vi "MouseMove.vi"(7 "Buffer":refnum<queue>, 8 "error in":errorcluster, 9 "Coords":T5, 11 "Data in":T1={"Class"={"Ants"=refnum, "Layer"=refnum, "Templates"=refnum, "Icon"=refnum, "Glyph"=refnum, "Settings"=refnum, "Tools"=refnum}, "Ref"={"Add Layer"=refnum, "Remove Layer"=refnum, "Line Text"=[], "Body Text Spec"=refnum, "DNL_Font"=refnum, "glyph path str"=refnum, "templates path str"=refnum, "Arrow Up"=refnum, "Arrow Down"=refnum, "IE VI Ref"=refnum, "Glyphs tree"=refnum, "Templates tree"=refnum, "Layer Icon Text"=refnum, "Layer Template"=refnum, "Body Text"=refnum, "Search Templates"=refnum, "TextMarker"=refnum, "Tab Control"=refnum, "Search Glyphs"=refnum, "Line Color"=refnum, "DNL_Glyphs []"=refnum, "Fill Color"=refnum, "Tools"=refnum, "Icon"=refnum, "Preview"=refnum, "Ants"=refnum, "Terminals"=refnum, "menu reference"=refnum, "LayerNames"=[], "GlyphLoadAnimation"=refnum, "TemplateLoadAnimation"=refnum, "refreshGlyphs"=refnum, "refreshTemplates"=refnum}, "Support"={"AntsRect"={"left"=0, "top"=0, "right"=0, "bottom"=0}, "Mouse Move Coords"={"Horizontal"=0, "Vertical"=0}, "Mouse Down Coords"={"Horizontal"=0, "Vertical"=0}, "Temp Coord"={"Horizontal"=0, "Vertical"=0}, "Action"=enum."Default", "Edge Color"=4914962, "Fill Color"=16860, "Mouse Down?"=FALSE, "Draft Mode?"=FALSE, "Temp Icon"=bytes[3102], "CTRL Pressed"=FALSE, "Move Selection?"=FALSE, "AntsRect Orig"={"left"=0, "top"=0, "right"=0, "bottom"=0}, "Text"="", "TM Set?"=FALSE, "Mouse inside icon?"=FALSE, "Tool (old value)"=0, "Pencil Move Color"=0, "Swap Colors?"=FALSE, "Shift pressed?"=FALSE}}) -> (0 "error out":errorcluster, 3 "Data out":T1={"Class"={"Ants"=refnum, "Layer"=refnum, "Templates"=refnum, "Icon"=refnum, "Glyph"=refnum, "Settings"=refnum, "Tools"=refnum}, "Ref"={"Add Layer"=refnum, "Remove Layer"=refnum, "Line Text"=[], "Body Text Spec"=refnum, "DNL_Font"=refnum, "glyph path str"=refnum, "templates path str"=refnum, "Arrow Up"=refnum, "Arrow Down"=refnum, "IE VI Ref"=refnum, "Glyphs tree"=refnum, "Templates tree"=refnum, "Layer Icon Text"=refnum, "Layer Template"=refnum, "Body Text"=refnum, "Search Templates"=refnum, "TextMarker"=refnum, "Tab Control"=refnum, "Search Glyphs"=refnum, "Line Color"=refnum, "DNL_Glyphs []"=refnum, "Fill Color"=refnum, "Tools"=refnum, "Icon"=refnum, "Preview"=refnum, "Ants"=refnum, "Terminals"=refnum, "menu reference"=refnum, "LayerNames"=[], "GlyphLoadAnimation"=refnum, "TemplateLoadAnimation"=refnum, "refreshGlyphs"=refnum, "refreshTemplates"=refnum}, "Support"={"AntsRect"={"left"=0, "top"=0, "right"=0, "bottom"=0}, "Mouse Move Coords"={"Horizontal"=0, "Vertical"=0}, "Mouse Down Coords"={"Horizontal"=0, "Vertical"=0}, "Temp Coord"={"Horizontal"=0, "Vertical"=0}, "Action"=enum."Default", "Edge Color"=4914962, "Fill Color"=16860, "Mouse Down?"=FALSE, "Draft Mode?"=FALSE, "Temp Icon"=bytes[3102], "CTRL Pressed"=FALSE, "Move Selection?"=FALSE, "AntsRect Orig"={"left"=0, "top"=0, "right"=0, "bottom"=0}, "Text"="", "TM Set?"=FALSE, "Mouse inside icon?"=FALSE, "Tool (old value)"=0, "Pencil Move Color"=0, "Swap Colors?"=FALSE, "Shift pressed?"=FALSE}})   [LabVIEW 2020]
uses:
  Class/Ants/Ants.lvclass
  Class/FakedArray/FakedArray.lvclass
  vi.lib/LabVIEW Icon API/lv_icon/Classes/Icon/Icon.lvclass
  Class/Icon Library/Glyph.lvclass
  Class/Settings/Settings.lvclass
  Class/Tools/Tools Paint.lvclass
  Controls/SupportClass_Action.ctl
  vi.lib/LabVIEW Icon API/lv_icon/lv_icon.lvlib
  <vilib>/Utility/miscctls.llb/LVPoint32TypeDef.ctl
  vi.lib/LabVIEW Icon API/lv_icon/Controls/IEColor.ctl
  Controls/SupportClass.ctl
  Controls/References Cluster.ctl
  Controls/IE Classes.ctl
  Controls/Global Data.ctl
panel:
  out "size(s)":i32
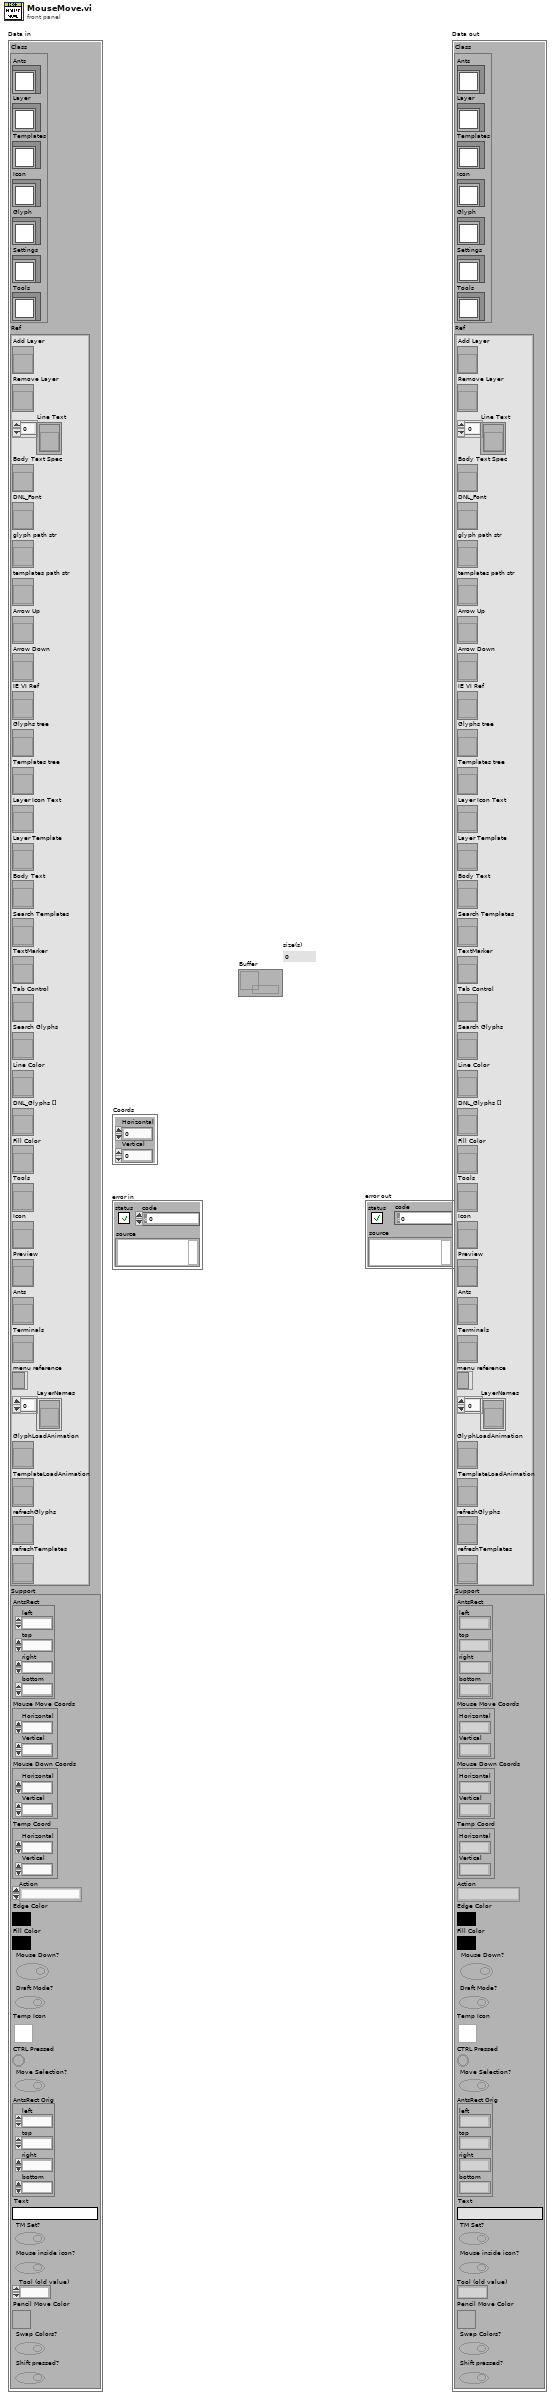
[diagram p1: front panel]
types:
  T1 = typedef "lv_icon.lvlib/Global Data.ctl" = cluster{"Class":T2, "Ref":T3, "Support":T4}
  T2 = typedef "IE Classes.ctl" = cluster{"Ants":refnum<class "Ants.lvclass">, "Layer":refnum<class "FakedArray.lvclass">, "Templates":refnum<class "FakedArray.lvclass">, "Icon":refnum<class "Icon.lvclass">, "Glyph":refnum<class "Glyph.lvclass">, "Settings":refnum<class "Settings.lvclass">, "Tools":refnum<class "Tools Paint.lvclass">}
  T3 = typedef "lv_icon.lvlib/References Cluster.ctl" = cluster{"Add Layer":refnum<vi>, "Remove Layer":refnum<vi>, "Line Text":refnum<vi>[], "Body Text Spec":refnum<vi>, "DNL_Font":refnum<vi>, "glyph path str":refnum<vi>, "templates path str":refnum<vi>, "Arrow Up":refnum<vi>, "Arrow Down":refnum<vi>, "IE VI Ref":refnum<vi>, "Glyphs tree":refnum<vi>, "Templates tree":refnum<vi>, "Layer Icon Text":refnum<vi>, "Layer Template":refnum<vi>, "Body Text":refnum<vi>, "Search Templates":refnum<vi>, "TextMarker":refnum<vi>, "Tab Control":refnum<vi>, "Search Glyphs":refnum<vi>, "Line Color":refnum<vi>, "DNL_Glyphs []":refnum<vi>, "Fill Color":refnum<vi>, "Tools":refnum<vi>, "Icon":refnum<vi>, "Preview":refnum<vi>, "Ants":refnum<vi>, "Terminals":refnum<vi>, "menu reference":refnum<k9>, "LayerNames":refnum<vi>[], "GlyphLoadAnimation":refnum<vi>, "TemplateLoadAnimation":refnum<vi>, "refreshGlyphs":refnum<vi>, "refreshTemplates":refnum<vi>}
  T4 = typedef "SupportClass.ctl" = cluster{"AntsRect":cluster{"left":i16, "top":i16, "right":i16, "bottom":i16}, "Mouse Move Coords":T5, "Mouse Down Coords":T5, "Temp Coord":T5, "Action":T6, "Edge Color":T7, "Fill Color":T7, "Mouse Down?":bool, "Draft Mode?":bool, "Temp Icon":picture, "CTRL Pressed":bool, "Move Selection?":bool, "AntsRect Orig":cluster{"left":i16, "top":i16, "right":i16, "bottom":i16}, "Text":string, "TM Set?":bool, "Mouse inside icon?":bool, "Tool (old value)":u32, "Pencil Move Color":u32, "Swap Colors?":bool, "Shift pressed?":bool}
  T5 = typedef "LVPoint32TypeDef.ctl" = cluster{"Horizontal":i32, "Vertical":i32}
  T6 = typedef "SupportClass_Action.ctl" = enum16{"Default", "Move Selection", "Glyph Library", "Tool"}
  T7 = typedef "IEColor.ctl" = u32
  T8 = cluster{"left":i16, "top":i16, "right":i16, "bottom":i16}
  T9 = typedef "Graphic.ctl" = cluster{"Rectangle":cluster{"left":i16, "top":i16, "right":i16, "bottom":i16}, "Path":path, "Image":picture, "Filter":string, "FileName":string}
  T10 = typedef "Tools.ctl" = enum32{"Pencil", "Line", "Dropper", "Fill", "Rectangle", "Filled Rectangle", "Ellipse", "Filled Ellipse", "Eraser", "Text", "Select", "Move"}
  T11 = cluster{"Horizontal":i32, "Vertical":i32, "Horizontal":i32, "Vertical":i32}
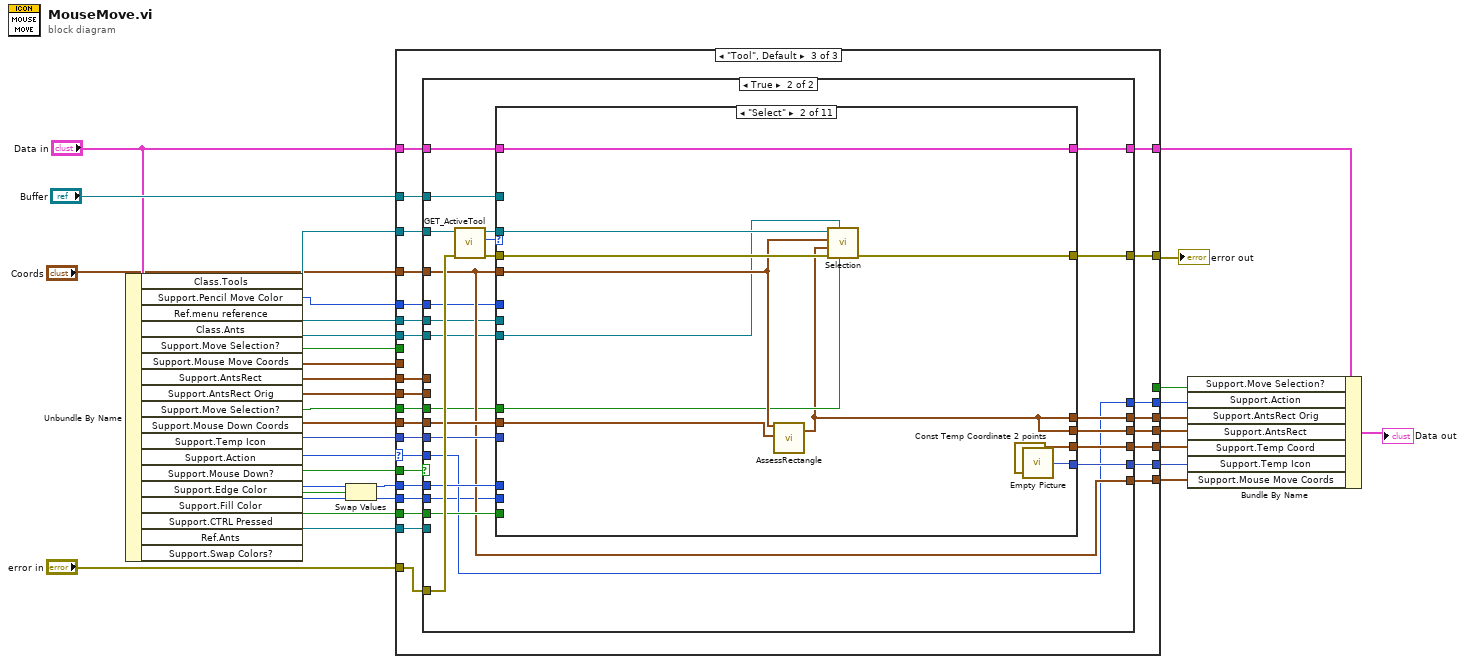
[diagram p0: block diagram]
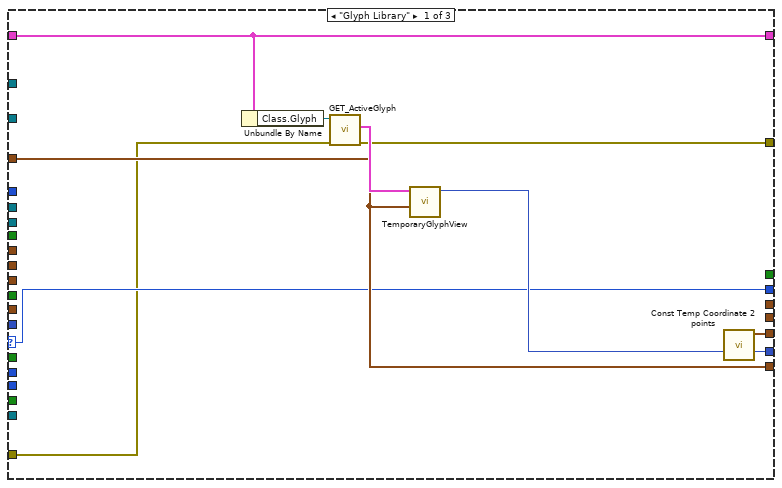
[diagram p2: hidden frame]
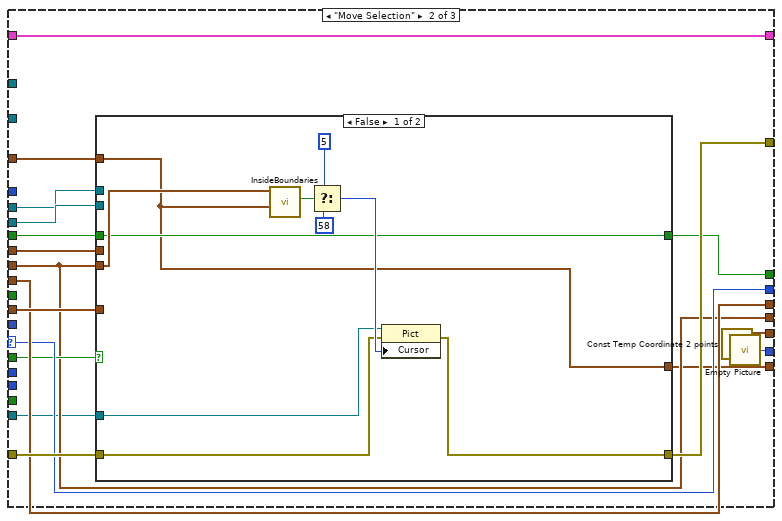
[diagram p3: hidden frame]
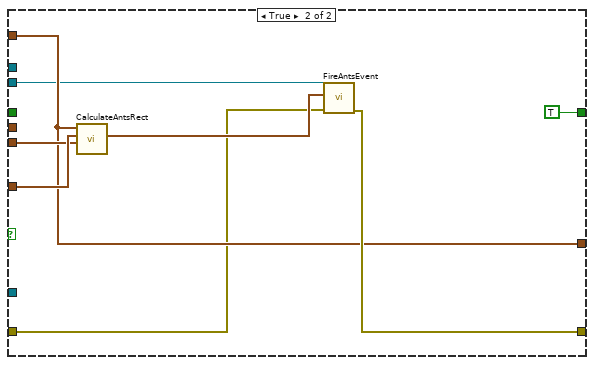
[diagram p4: hidden frame]
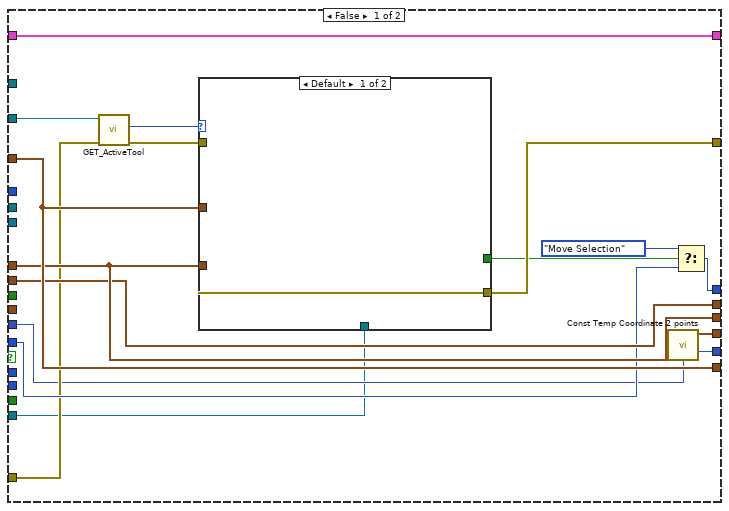
[diagram p5: hidden frame]
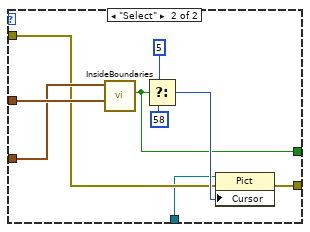
[diagram p6: hidden frame]
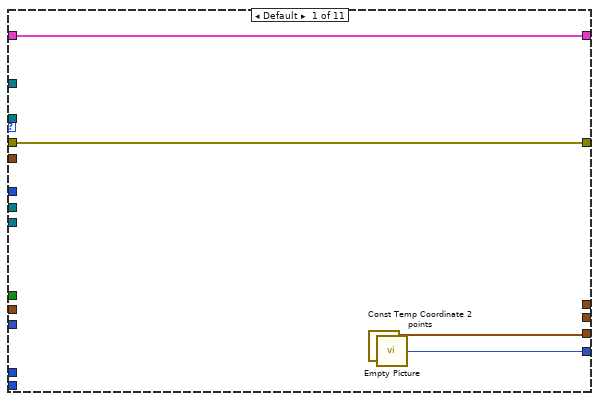
[diagram p7: hidden frame]
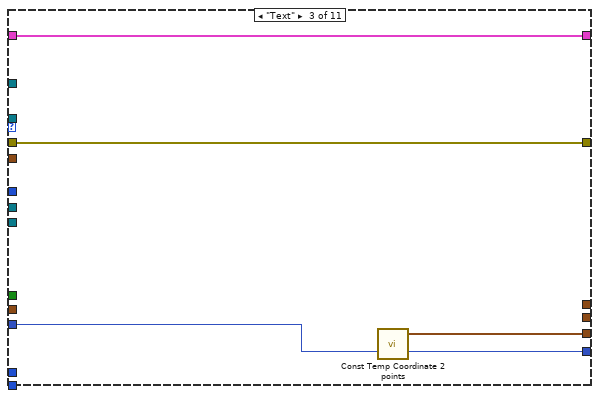
[diagram p8: hidden frame]
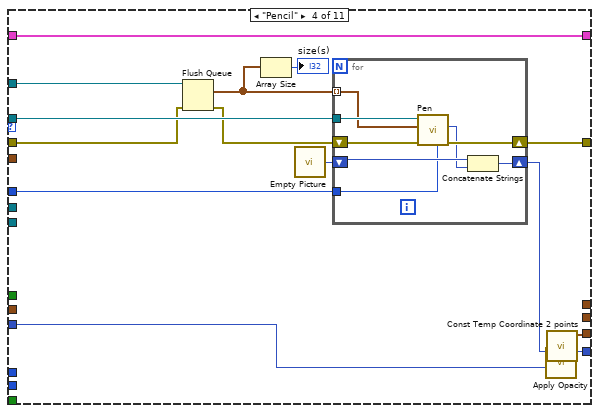
[diagram p9: hidden frame]
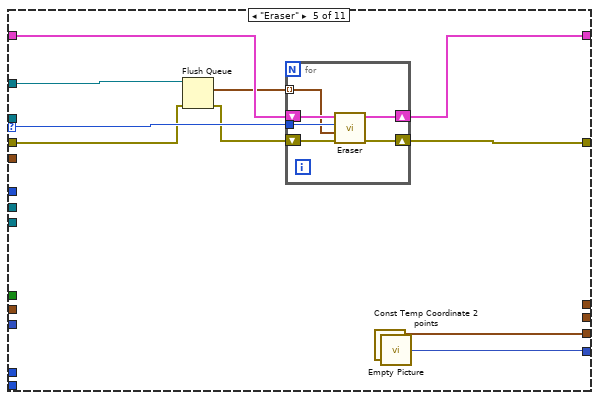
[diagram p10: hidden frame]
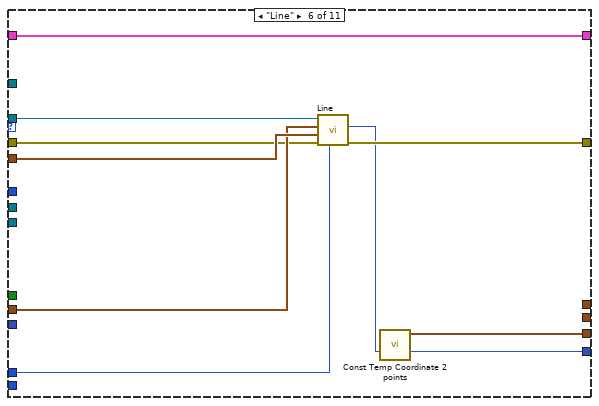
[diagram p11: hidden frame]
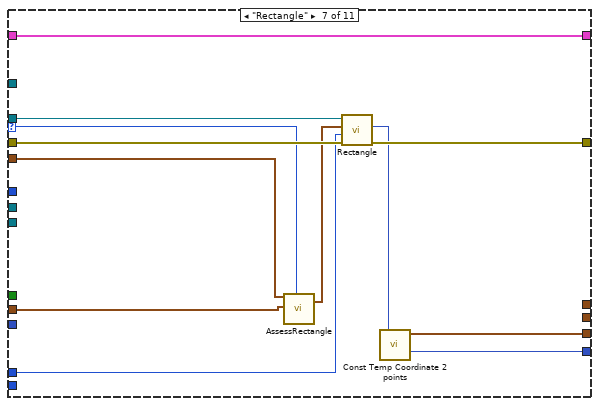
[diagram p12: hidden frame]
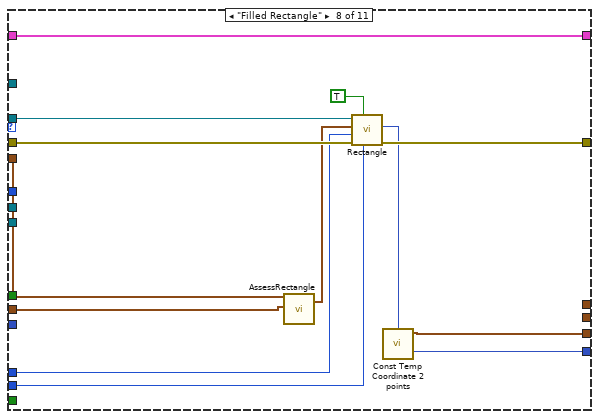
[diagram p13: hidden frame]
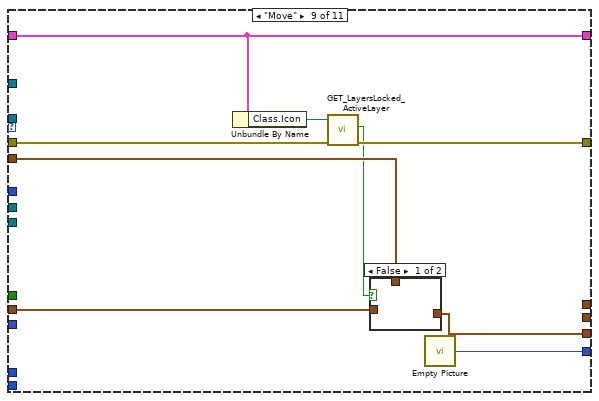
[diagram p14: hidden frame]
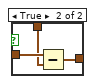
[diagram p15: hidden frame]
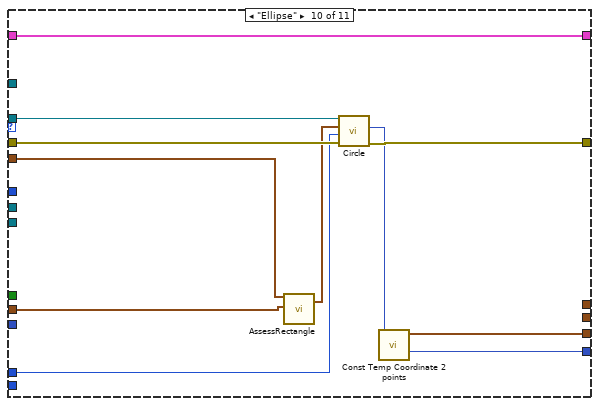
[diagram p16: hidden frame]
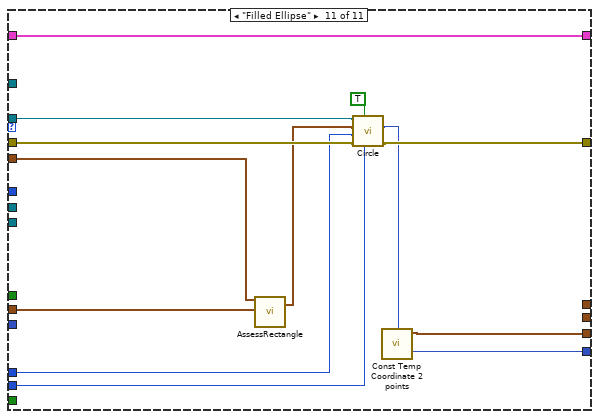
[diagram p17: hidden frame]
diagram:
  n1 = Unbundle By Name("Data in") -> ("Class.Tools"=w8:refnum<class "Tools Paint.lvclass">, "Support.Pencil Move Color"=w7:u32, "Ref.menu reference"=w9:refnum<k9>, "Class.Ants"=w10:refnum<class "Ants.lvclass">, "Support.Move Selection?"=w18:bool, "Support.Mouse Move Coords"=w19:T5, "Support.AntsRect"=w22:T8, "Support.AntsRect Orig"=w24:T8, "Support.Move Selection?"=w26:bool, "Support.Mouse Down Coords"=w30:T5, "Support.Temp Icon"=w28:picture, "Support.Action"=w27:T6, "Support.Mouse Down?"=w29:bool, "Support.Edge Color"=w6:T7, "Support.Fill Color"=w4:T7, "Support.CTRL Pressed"=w31:bool, "Ref.Ants"=w11:refnum<vi>, "Support.Swap Colors?"=w2:bool)
  n2 = Swap Values(12:w6, 13:w2, 14:w4) -> (1:w5:T7, 3:w3:T7)
  n3 = case shown="\"Tool\", Default" w27 {
    selector: w27 -> [w38 w54 w90]
    tunnel: "Coords" -> [w40 w57 w104]
    tunnel: "error in" -> [w37 w59 w106]
    tunnel: [w42 w58 w103] -> w14
    tunnel: w28 -> [_ _ w105]
    tunnel: w29 -> [_ w53 w102]
    tunnel: w30 -> [_ w56 w101]
    tunnel: w5 -> [_ _ w100]
    tunnel: w31 -> [_ _ w99]
    tunnel: [w41 w60 w98] -> w32
    tunnel: [w40 w49 w97] -> w33
    tunnel: [w39 w61 w96] -> w34
    tunnel: w26 -> [_ _ w95]
    tunnel: [_ w51 w94] -> w25
    tunnel: w24 -> [_ w55 w93]
    tunnel: [_ w55 w92] -> w23
    tunnel: w22 -> [_ w51 w91]
    tunnel: [w38 w54 w89] -> w21
    tunnel: [_ w52 _] -> w20
    tunnel: w19 -> [_ w50 _]
    tunnel: w18 -> [_ w48 _]
    tunnel: w3 -> [_ _ w88]
    tunnel: w8 -> [_ _ w87]
    tunnel: "Buffer" -> [_ _ w86]
    tunnel: "Data in" -> [w35 w45 w85]
    tunnel: [w35 w45 w84] -> w12
    tunnel: w11 -> [_ w47 w83]
    tunnel: w10 -> [_ w46 w82]
    tunnel: w9 -> [_ w44 w81]
    tunnel: w7 -> [_ _ w80]
    frame "Glyph Library" {
      n4 = Unbundle By Name(w35) -> ("Class.Glyph"=w36:refnum<class "Glyph.lvclass">)
      n5 = call-dynamic "GET_ActiveGlyph.vi"("error in (no error)"=w37, "Glyph.lvclass in"=w36) -> ("error out"=w42:errorcluster, "Path & Icon"=w43:T9)  [unwired: 8 out]
      n6 = call "TemporaryGlyphView.vi"("Mouse Coords Pic"=w40, "Path & Icon"=w43) -> ("icon out"=w41:picture)  [unwired: 9 out]
      n7 = call "Const Temp Coordinate 2 points.vi"() -> ("Const Temp Coordinate"=w39:T5)  [unwired: 11 out]
    }
    frame "Move Selection" {
      n8 = case shown="False" w53 {
        tunnel: w59 -> [w63 w73]
        tunnel: [w67 w79] -> w58
        tunnel: w57 -> [w64 w74]
        tunnel: w56 -> [_ w77]
        tunnel: w51 -> [w66 w76]
        tunnel: [w65 TRUE] -> w52
        tunnel: w50 -> [_ _]
        tunnel: [w64 w74] -> w49
        tunnel: w48 -> [w65 _]
        tunnel: w47 -> [w62 _]
        tunnel: w46 -> [_ w72]
        tunnel: w44 -> [_ _]
        frame False {
          n9 = call "InsideBoundaries.vi"("Mouse Move Coords"=w64, "AntsRect"=w66) -> ("Inside?"=w68:bool)  [unwired: 9 out]
          n10 = Select(t=5 ("Cursor"), s=w68, f=58 ("Cursor")) -> (s? t:f=w69:i32)
          n11 = property class="Pict"(reference=w62, error in=w63, "Cursor"=w69) -> (error out=w67:errorcluster)  [unwired: 1 out]
        }
        frame True {
          n12 = call "CalculateAntsRect.vi"("AntsRect"=w76, "Mouse Down Coords"=w77, "Mouse Move Coords"=w74) -> ("Rect"=w75:cluster{i32, i32, i32, i32})  [unwired: 8 out]
          n13 = call "FireAntsEvent.vi"("error in (no error)"=w73, "Rectangle (default: deselect)"=w75, "Ants in"=w72) -> ("error out"=w79:errorcluster)  [unwired: 1 in, 7 out]
        }
      }
      n14 = call "Const Temp Coordinate 2 points.vi"() -> ("Const Temp Coordinate"=w61:T5)  [unwired: 11 out]
      n15 = call "Empty Picture"() -> ("empty picture"=w60:picture)
    }
    frame "Tool", Default {
      n16 = case shown="True" w102 {
        tunnel: w106 -> [w110 w156]
        tunnel: w105 -> [w109 w153]
        tunnel: w104 -> [w119 w146]
        tunnel: [w118 w151] -> w103
        tunnel: w101 -> [_ w150]
        tunnel: w100 -> [_ w149]
        tunnel: w99 -> [_ w148]
        tunnel: [w109 w147] -> w98
        tunnel: [w119 w146] -> w97
        tunnel: [w122 w145] -> w96
        tunnel: w95 -> [_ w144]
        tunnel: [w117 w143] -> w94
        tunnel: w93 -> [w116 _]
        tunnel: [w116 w142] -> w92
        tunnel: w91 -> [w117 _]
        tunnel: w90 -> [w114 w141]
        tunnel: [w112 w141] -> w89
        tunnel: w88 -> [_ w140]
        tunnel: w87 -> [w111 w139]
        tunnel: w86 -> [_ w138]
        tunnel: w85 -> [w107 w134]
        tunnel: [w107 w137] -> w84
        tunnel: w83 -> [w108 _]
        tunnel: w82 -> [_ w136]
        tunnel: w81 -> [_ w135]
        tunnel: w80 -> [_ w133]
        frame False {
          n17 = call-dynamic "GET_ActiveTool.vi"("error in (no error)"=w110, "Tools Paint.lvclass in"=w111) -> ("error out"=w121:errorcluster, "Radio Buttons"=w120:T10)  [unwired: 8 out]
          n18 = case shown="Default" w120 {
            tunnel: w121 -> [w123 w125]
            tunnel: w119 -> [_ w129]
            tunnel: [w123 w128] -> w118
            tunnel: w117 -> [_ w127]
            tunnel: [_ w126] -> w115
            tunnel: w108 -> [_ w124]
            frame Default {
            }
            frame "Select" {
              n19 = call "InsideBoundaries.vi"("Mouse Move Coords"=w129, "AntsRect"=w127) -> ("Inside?"=w126:bool)  [unwired: 9 out]
              n20 = Select(t=5 ("Cursor"), s=w126, f=58 ("Cursor")) -> (s? t:f=w130:i32)
              n21 = property class="Pict"(reference=w124, error in=w125, "Cursor"=w130) -> (error out=w128:errorcluster)  [unwired: 1 out]
            }
          }
          n22 = call "Const Temp Coordinate 2 points.vi"() -> ("Const Temp Coordinate"=w122:T5)  [unwired: 11 out]
          n23 = Select(t=SupportClass_Action."Move Selection", s=w115, f=w114) -> (s? t:f=w112:T6)
        }
        frame True {
          n24 = call-dynamic "GET_ActiveTool.vi"("error in (no error)"=w156, "Tools Paint.lvclass in"=w139) -> ("error out"=w154:errorcluster, "Radio Buttons"=w155:T10, "Tools Paint.lvclass out"=w152:refnum<class "Tools Paint.lvclass">)  [unwired: 7 out]
          n25 = case shown="\"Select\"" w155 {
            selector: w155 -> [_ _ _ _ w205 _ w225 _ _ _ _]
            tunnel: w154 -> [w160 w171 w175 w179 w200 w219 w232 w244 w248 w264 w276]
            tunnel: w153 -> [_ _ w174 w181 _ _ _ _ _ _ _]
            tunnel: w152 -> [_ w169 _ w189 _ w222 w233 w245 _ w265 w277]
            tunnel: w146 -> [_ w167 _ _ _ w221 w229 w241 w251 w267 w279]
            tunnel: w149 -> [_ _ _ _ _ w216 w226 w238 _ w260 w272]
            tunnel: [w160 w170 w175 w188 w207 w218 w231 w243 w250 w263 w275] -> w151
            tunnel: [w159 w164 w174 w187 w206 w217 w230 w242 w252 w262 w274] -> w147
            tunnel: w150 -> [_ w168 _ _ _ w220 w228 w240 w254 w266 w278]
            tunnel: w148 -> [_ _ _ _ _ _ _ _ _ _ _]
            tunnel: [w158 w165 w173 w186 w204 w215 w224 w237 w253 w259 w271] -> w145
            tunnel: w144 -> [_ w166 _ _ _ _ _ _ _ _ _]
            tunnel: [_ w163 _ _ _ _ _ _ _ _ _] -> w143
            tunnel: [_ w163 _ _ _ _ _ _ _ _ _] -> w142
            tunnel: w140 -> [_ _ _ _ _ _ _ w234 _ _ w268]
            tunnel: w138 -> [_ _ _ w185 w201 _ _ _ _ _ _]
            tunnel: w134 -> [w157 w162 w172 w180 w203 w214 w223 w235 w246 w258 w269]
            tunnel: [w157 w162 w172 w180 w202 w214 w223 w235 w246 w258 w269] -> w137
            tunnel: w136 -> [_ w161 _ _ _ _ _ _ _ _ _]
            tunnel: w135 -> [_ _ _ _ _ _ _ _ _ _ _]
            tunnel: w133 -> [_ _ _ w178 _ _ _ _ _ _ _]
            frame Default {
              n26 = call "Const Temp Coordinate 2 points.vi"() -> ("Const Temp Coordinate"=w158:T5)  [unwired: 11 out]
              n27 = call "Empty Picture"() -> ("empty picture"=w159:picture)
            }
            frame "Select" {
              n28 = call "AssessRectangle.vi"("Coords In 1"=w167, "Coords In 2"=w168) -> ("Rectangle"=w163:T11)  [unwired: 1 in, 16 out]
              n29 = call "Selection.vi"("Move Selection?"=w166, "Ants"=w161, "error in (no error)"=w171, "Ants Selection"=w163, "Current Coords"=w167, "Tools Paint in"=w169) -> ("error out"=w170:errorcluster)  [unwired: 1 in, 4 out]
              n30 = call "Const Temp Coordinate 2 points.vi"() -> ("Const Temp Coordinate"=w165:T5)  [unwired: 11 out]
              n31 = call "Empty Picture"() -> ("empty picture"=w164:picture)
            }
            frame "Text" {
              n32 = call "Const Temp Coordinate 2 points.vi"() -> ("Const Temp Coordinate"=w173:T5)  [unwired: 11 out]
            }
            frame "Pencil" {
              n33 = Flush Queue(queue=w185, error in (no error)=w179) -> (remaining elements=w177:T5[], error out=w184:errorcluster)  [unwired: 1 out]
              n34 = Array Size(array=w177) -> (size(s)=→"size(s)":i32)
              n35 = call "Empty Picture"() -> ("empty picture"=w183:picture)
              n36 = for {
                tunnel: w189 -> [w197]
                shift-right: [w196] -> w188
                shift-left: w184 -> [w195]
                tunnel: w177 -> [w191] mode=indexing
                shift-right: [w192] -> w182
                shift-left: w183 -> [w194]
                tunnel: w178 -> [w190]
                n37 = call-dynamic "Pen.vi"("Edge color"=w190, "error in (no error)"=w195, "point(x,y)"=w191, "Tools Paint in"=w197) -> ("error out"=w196:errorcluster, "new picture"=w193:picture)  [unwired: 2 in, 4 out]
                n38 = Concatenate Strings(w194, w193) -> (w192:picture)
              }
              n39 = call "Apply Opacity.vi"("Bottom"=w181, "Top"=w182) -> ("new picture"=w187:picture)  [unwired: 1 in, 8 out]
              n40 = call "Const Temp Coordinate 2 points.vi"() -> ("Const Temp Coordinate"=w186:T5)  [unwired: 11 out]
            }
            frame "Eraser" {
              n41 = Flush Queue(queue=w201, error in (no error)=w200) -> (remaining elements=w198:T5[], error out=w199:errorcluster)  [unwired: 1 out]
              n42 = for {
                tunnel: w205 -> [w211]
                shift-right: [w209] -> w202
                shift-left: w203 -> [w210]
                tunnel: w198 -> [w208] mode=indexing
                shift-right: [w213] -> w207
                shift-left: w199 -> [w212]
                n43 = call "Eraser.vi"("error in (no error)"=w212, "point(x,y)"=w208, "Radio Buttons"=w211, "Data in"=w210) -> ("error out"=w213:errorcluster, "Data out"=w209:T1)  [unwired: 6 out]
              }
              n44 = call "Const Temp Coordinate 2 points.vi"() -> ("Const Temp Coordinate"=w204:T5)  [unwired: 11 out]
              n45 = call "Empty Picture"() -> ("empty picture"=w206:picture)
            }
            frame "Line" {
              n46 = call-dynamic "Line.vi"("color(black)"=w216, "error in (no error)"=w219, "end point"=w221, "new position"=w220, "Tools Paint in"=w222) -> ("error out"=w218:errorcluster, "new picture"=w217:picture)  [unwired: 5 out]
              n47 = call "Const Temp Coordinate 2 points.vi"() -> ("Const Temp Coordinate"=w215:T5)  [unwired: 11 out]
            }
            frame "Rectangle" {
              n48 = call "AssessRectangle.vi"("Coords In 1"=w229, "Coords In 2"=w228, "Tool"=w225) -> ("Rectangle"=w227:T11)  [unwired: 16 out]
              n49 = call-dynamic "Rectangle.vi"("error in (no error)"=w232, "Edge Color"=w226, "rect"=w227, "Tools Paint in"=w233) -> ("error out"=w231:errorcluster, "new picture"=w230:picture)  [unwired: 2 in, 4 out]
              n50 = call "Const Temp Coordinate 2 points.vi"() -> ("Const Temp Coordinate"=w224:T5)  [unwired: 11 out]
            }
            frame "Filled Rectangle" {
              n51 = call "AssessRectangle.vi"("Coords In 1"=w241, "Coords In 2"=w240) -> ("Rectangle"=w239:T11)  [unwired: 1 in, 16 out]
              n52 = call-dynamic "Rectangle.vi"("Fill Color"=w234, "fill?(F)"=TRUE, "error in (no error)"=w244, "Edge Color"=w238, "rect"=w239, "Tools Paint in"=w245) -> ("error out"=w243:errorcluster, "new picture"=w242:picture)  [unwired: 4 out]
              n53 = call "Const Temp Coordinate 2 points.vi"() -> ("Const Temp Coordinate"=w237:T5)  [unwired: 11 out]
            }
            frame "Move" {
              n54 = Unbundle By Name(w246) -> ("Class.Icon"=w247:refnum<class "Icon.lvclass">)
              n55 = call-dynamic "GET_LayersLocked_ActiveLayer.vi"("error in (no error)"=w248, "Icon.lvclass in"=w247) -> ("error out"=w250:errorcluster, "Layers Locked?"=w249:bool)  [unwired: 8 out]
              n56 = case shown="False" w249 {
                tunnel: w254 -> [_ w257]
                tunnel: [_ w256] -> w253
                tunnel: w251 -> [_ w255]
                frame False {
                }
                frame True {
                  n57 = Subtract(x=w257, y=w255) -> (x-y=w256:T5)
                }
              }
              n58 = call "Empty Picture"() -> ("empty picture"=w252:picture)
            }
            frame "Ellipse" {
              n59 = call "AssessRectangle.vi"("Coords In 1"=w267, "Coords In 2"=w266) -> ("Rectangle"=w261:T11)  [unwired: 1 in, 16 out]
              n60 = call-dynamic "Circle.vi"("error in (no error)"=w264, "Edge Color"=w260, "rect"=w261, "Tools Paint in"=w265) -> ("error out"=w263:errorcluster, "new picture"=w262:picture)  [unwired: 2 in, 4 out]
              n61 = call "Const Temp Coordinate 2 points.vi"() -> ("Const Temp Coordinate"=w259:T5)  [unwired: 11 out]
            }
            frame "Filled Ellipse" {
              n62 = call "AssessRectangle.vi"("Coords In 1"=w279, "Coords In 2"=w278) -> ("Rectangle"=w273:T11)  [unwired: 1 in, 16 out]
              n63 = call-dynamic "Circle.vi"("Fill Color"=w268, "fill?(F)"=TRUE, "error in (no error)"=w276, "Edge Color"=w272, "rect"=w273, "Tools Paint in"=w277) -> ("error out"=w275:errorcluster, "new picture"=w274:picture)  [unwired: 4 out]
              n64 = call "Const Temp Coordinate 2 points.vi"() -> ("Const Temp Coordinate"=w271:T5)  [unwired: 11 out]
            }
          }
        }
      }
    }
  }
  "error out" <- w14
  n65 = Bundle By Name(cluster=w12, "Support.Move Selection?"=w20, "Support.Action"=w21, "Support.AntsRect Orig"=w23, "Support.AntsRect"=w25, "Support.Temp Coord"=w34, "Support.Temp Icon"=w32, "Support.Mouse Move Coords"=w33) -> (→"Data out":T1)
